vi "create distribution plot hdf.vi"(4 "y bin":i32=100, 5 "y row":i32=4, 6 "x bin":i32=100, 7 "x row":i32=3, 8 "error in (no error)":errorcluster, 9 "length":i32, 10 "start":i32, 11 "Path":path=path "C:/Users/yg/Desktop/tmp/20230322-230510 test_readout.h5") -> (0 "error out":errorcluster, 2 "Cluster":T1, 3 "Intensity Graph":dbl[][](graph))   [LabVIEW 2021]
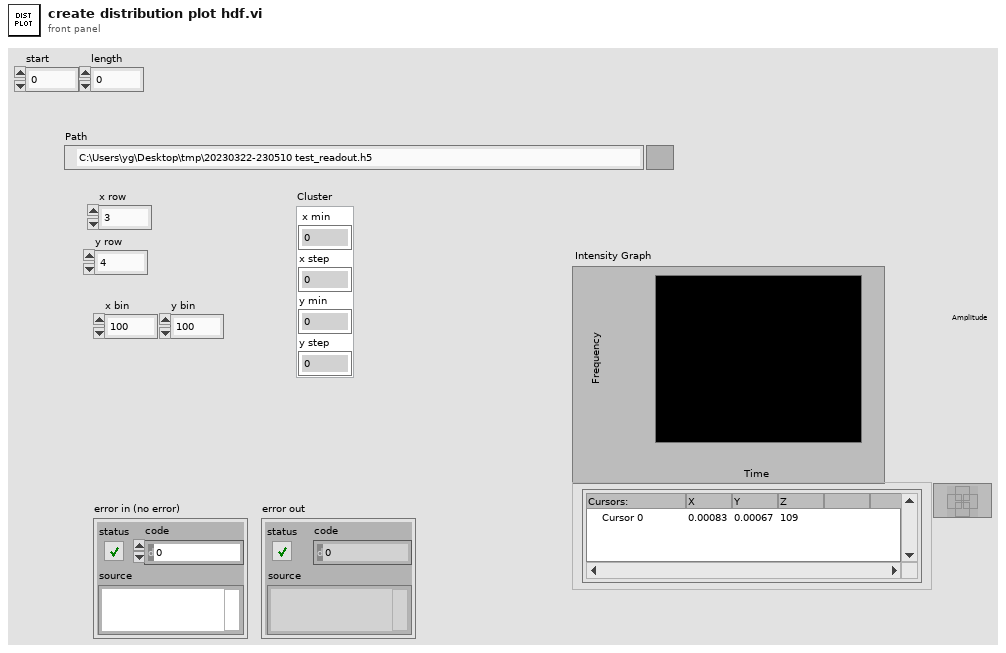
[diagram p1: front panel]
types:
  T1 = cluster{" x min":dbl, "x step":dbl, "y min":dbl, "y step":dbl}
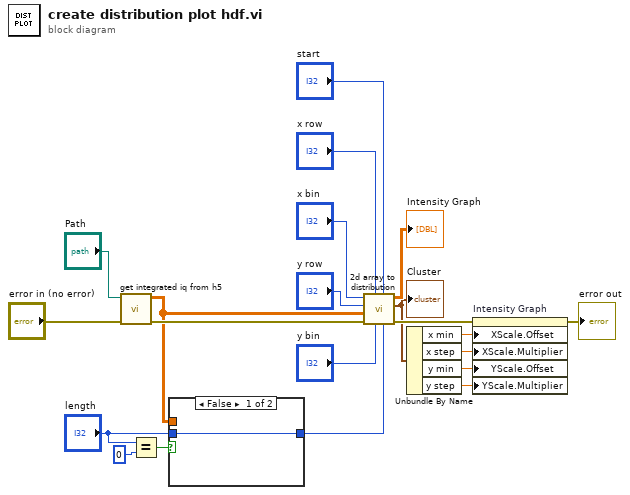
[diagram p0: block diagram]
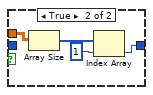
[diagram p2: hidden frame]
diagram:
  n1 = call "get integrated iq from h5.vi"("error in (no error)"="error in (no error)", "path"="Path") -> ("error out"=w7:errorcluster, "Data out"=w3:dbl[][])  [unwired: 8 in]
  n2 = Equal?(x="length", y=0) -> (x = y?=w4:bool)
  n3 = case shown="False" w4 {
    tunnel: w3 -> [_ w26]
    tunnel: [w22 w23] -> w2
    tunnel: "length" -> [w22 _]
    frame False {
    }
    frame True {
      n4 = Array Size(array=w26) -> (size(s)=w25:i32[])
      n5 = Index Array(array=w25, index=1) -> (element=w23:i32)
    }
  }
  n6 = call "2d array to distribution.vi"("length"=w2, "start"="start", "y bin"="y bin", "x row"="x row", "error in (no error)"=w7, "all rows"=w3, "y row"="y row", "x bin"="x bin") -> ("error out"=w20:errorcluster, "Cluster"=w19:T1, "Array"=→"Intensity Graph":dbl[][])  [unwired: 1 in]
  "Cluster" <- w19
  n7 = Unbundle By Name(w19) -> ("x min"=w18:dbl, "x step"=w17:dbl, "y min"=w16:dbl, "y step"=w15:dbl)
  n8 = property on="Intensity Graph" class="IntGraph (strict)"(error in=w20, "XScale.Offset"=w18, "XScale.Multiplier"=w17, "YScale.Offset"=w16, "YScale.Multiplier"=w15) -> (error out=→"error out":errorcluster)  [unwired: 1 in, 1 out]
